vi "turnanddrive.vi"(0 "RobotDriveDevRef":T1={"DevStatus"={"status"=FALSE, "code"=0, "source"=""}, "Motors[]"=[], "Square Inputs"=FALSE, "Max Output"=1.0}, 5 "y":i32=-1, 7 "distance":i32=100, 11 "Angle":dbl=45.0 format="%#_13g") -> (4 "RobotDriveDevRef dup.":T1={"DevStatus"={"status"=FALSE, "code"=0, "source"=""}, "Motors[]"=[], "Square Inputs"=FALSE, "Max Output"=1.0})   [LabVIEW 2016]
uses:
  <vilib>/Rock Robotics/WPI/RobotDrive/WPI_RobotDriveDevRef.ctl
  <vilib>/Rock Robotics/WPI/MotorControl/WPI_MotorControlDeviceRef.ctl
  <vilib>/Rock Robotics/WPI/MotorControl/WPI_MotorControlType.ctl
  <vilib>/Rock Robotics/SystemInterfaces/DIO/FPGA_DIOPWMChannel.ctl
  <vilib>/Rock Robotics/WPI/PWM/WPI_PWMDeadband.ctl
  <vilib>/Rock Robotics/WPI/RobotDrive/WPI_RobotDriveArcadeDrive_Standard(NoSaturation).vi
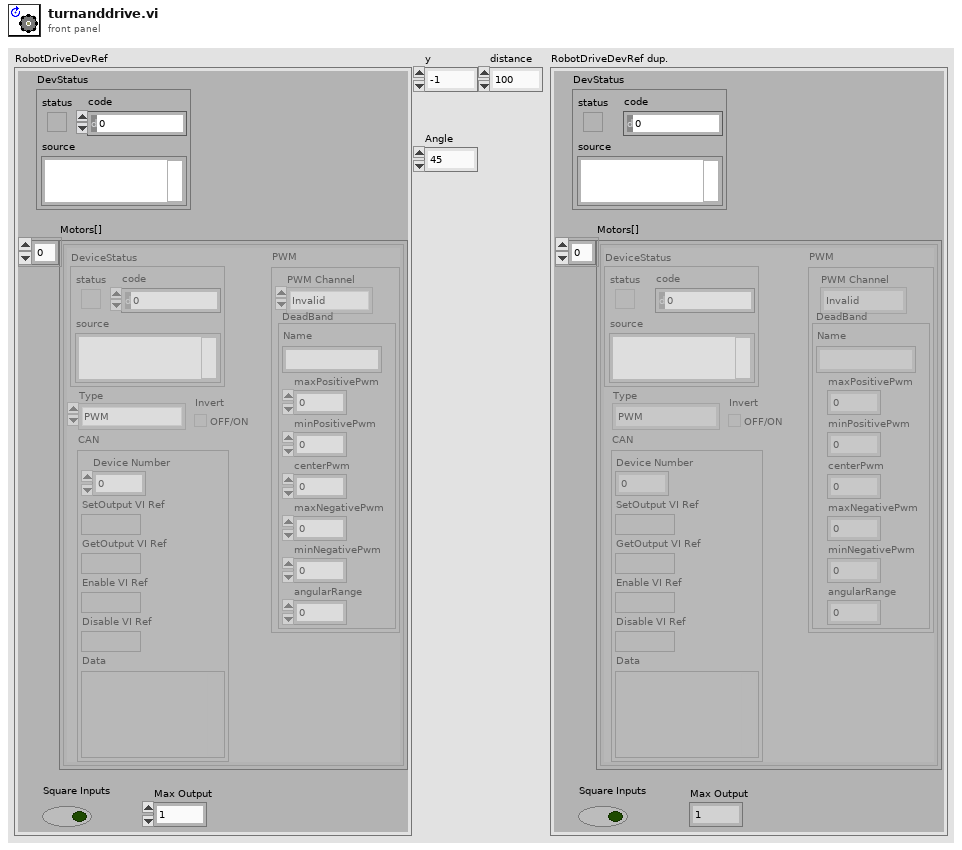
[diagram p1: front panel]
types:
  T1 = typedef "WPI_RobotDriveDevRef.ctl" = cluster{"DevStatus":errorcluster, "Motors[]":T2[], "Square Inputs":bool, "Max Output":dbl}
  T2 = typedef "WPI_MotorControlDeviceRef.ctl" = cluster{"DeviceStatus":errorcluster, "Type":T3, "PWM":cluster{"PWM Channel":T4, "DeadBand":T5}, "CAN":cluster{"Device Number":u8, "SetOutput VI Ref":variant, "GetOutput VI Ref":variant, "Enable VI Ref":variant, "Disable VI Ref":variant, "Data":variant}, "Invert":bool}
  T3 = typedef "WPI_MotorControlType.ctl" = enum16{"PWM", "CAN"}
  T4 = typedef "FPGA_DIOPWMChannel.ctl" = enum8{"PWM 0", "PWM 1", "PWM 2", "PWM 3", "PWM 4", "PWM 5", "PWM 6", "PWM 7", "PWM 8", "PWM 9", "PWM MXP 0", "PWM MXP 1", "PWM MXP 2", "PWM MXP 3", "PWM MXP 4", "PWM MXP 5", "PWM MXP 6", "PWM MXP 7", "PWM MXP 8", "PWM MXP 9", "Invalid"}
  T5 = typedef "WPI_PWMDeadband.ctl" = cluster{"Name":string, "maxPositivePwm":i32, "minPositivePwm":i32, "centerPwm":i32, "maxNegativePwm":i32, "minNegativePwm":i32, "angularRange":u16}
  T6 = typedef "WPI_GyroDevRef.ctl" = cluster{"DevStatus":errorcluster, "Analog Channel":T7, "Offset":dbl, "Gain (VoltsPerDegree/Second)":dbl, "Gyro Type":enum16{"Analog", "XRS450"}, "Handle":i32, "SPI Bus":T8, "Device Found":bool, "Sample Rate":dbl, "Calibrate On Open":bool}
  T7 = typedef "FPGA_AIChannel.ctl" = enum8{"AI 0", "AI 1", "AI 2", "AI 3", "AI MXP 0", "AI MXP 1", "AI MXP 2", "AI MXP 3", "Invalid"}
  T8 = typedef "spi_bus.ctl" = enum16{"SPI On-Board, CS0", "SPI On-Board, CS1", "SPI On-Board, CS2", "SPI On-Board, CS3", "SPI MXP", "Invalid"}
  T9 = typedef "WPI_CANJaguar_Status.ctl" = cluster{"Output Percent VBus":dbl, "Output Voltage":dbl, "Bus Voltage":dbl, "Current":dbl, "Temperature":dbl, "Position":dbl, "Speed":dbl, "Limits":cluster{"Forward Limit":bool, "Reverse Limit":bool, "Forward Soft Limit":bool, "Reverse Soft Limit":bool, "Sticky Forward Limit":bool, "Sticky Reverse Limit":bool, "Sticky Forward Soft Limit":bool, "Sticky Reverse Soft Limit":bool}, "Faults":cluster{"Current Fault":bool, "Temperature Fault":bool, "Bus Voltage Fault":bool, "Gate Driver Fault":bool, "Comm Fault":bool}, "Fault Counters":cluster{"Current Faults":u8, "Temperature Faults":u8, "Bus Voltage Faults":u8, "Gate Driver Faults":u8, "Comm Faults":u8, "CAN Status":u8, "CAN RX Errors":u8, "CAN TX Errors":u8}, "Power Cycle":bool}
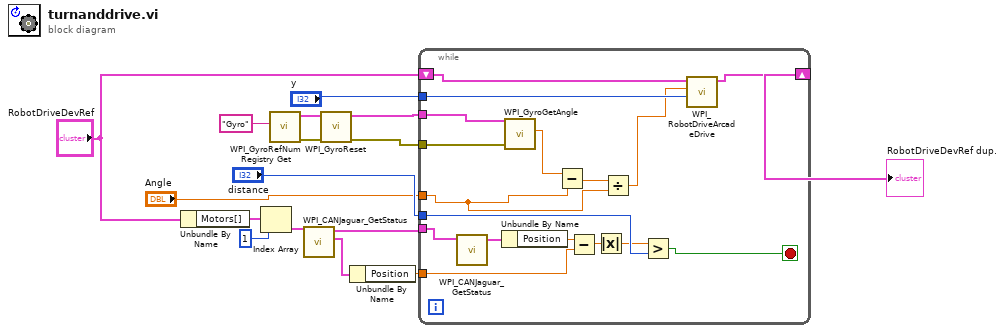
[diagram p0: block diagram]
diagram:
  n1 = Unbundle By Name("RobotDriveDevRef") -> ("Motors[]"=w16:T2[])
  n2 = Index Array(array=w16, index=1) -> (element=w5:T2)
  n3 = call <vilib>:"WPI_GyroRefNum Registry Get.vi"("refnum name"="Gyro") -> ("error out"=w7:errorcluster, "GyroDevRef"=w9:T6)  [unwired: 9 in]
  n4 = call <vilib>:"WPI_CANJaguar_GetStatus.vi"("CAN Jaguar Ref"=w5) -> ("Status"=w2:T9, "CAN Jaguar Ref"=w3:T2)  [unwired: 8 in, 1 out]
  n5 = call <vilib>:"WPI_GyroReset.vi"("error in"=w7, "GyroDevRef"=w9) -> ("error out"=w6:errorcluster, "GyroDevRef"=w8:T6)  [unwired: 8 in]
  n6 = Unbundle By Name(w2) -> ("Position"=w1:dbl)
  n7 = while {
    shift-right: [w32] -> w14
    shift-left: "RobotDriveDevRef" -> [w33]
    tunnel: w3 -> [w20]
    tunnel: "y" -> [w30]
    tunnel: "distance" -> [w29]
    tunnel: "Angle" -> [w28]
    tunnel: w6 -> [w23]
    tunnel: w8 -> [w22]
    tunnel: w1 -> [w17]
    stop <- w26 stop-if-true
    n8 = call <vilib>:"WPI_CANJaguar_GetStatus.vi"("CAN Jaguar Ref"=w20) -> ("Status"=w21:T9)  [unwired: 8 in, 2 out]
    n9 = Unbundle By Name(w21) -> ("Position"=w19:dbl)
    n10 = call <vilib>:"WPI_GyroGetAngle.vi"("error in"=w23, "GyroDevRef"=w22) -> ("Angle"=w24:dbl)  [unwired: 5 in, 4 out]
    n11 = Subtract(x=w24, y=w28) -> (x-y=w31:dbl)
    n12 = Subtract(x=w19, y=w17) -> (x-y=w18:dbl)
    n13 = Absolute Value(x=w18) -> (abs(x)=w27:dbl)
    n14 = Divide(x=w31, y=w28) -> (x/y=w25:dbl)
    n15 = Greater?(x=w27, y=w29) -> (0:w26:bool)
    n16 = call-poly <vilib>:"WPI_RobotDriveArcadeDrive.vi"("Y axis value"=w30, "X axis value"=w25, "RobotDriveDevRef"=w33) -> ("RobotDriveDevRef"=w32:T1)  [unwired: 6 in, 2 out]
  }
  "RobotDriveDevRef dup." <- w14
